vi "Auto_Routine_RightTwoPieceThen2CenterTRAJ.vi"   [LabVIEW 2023]
uses:
  Arm2/ArmGetSetpointEnum.ctl
  Trajectory/TrajectoryGlobals.vi
  <vilib>/Rock Robotics/WPI/ThirdParty/JAS_Junk/TrajLib/Trajectory_Library.lvlib
types:
  T1 = typedef "ArmGetSetpointEnum.ctl" = enum16{"ArmFloorPickup", "ArmAmpDeposit", "ArmSpeakerShoot", "ArmStartPosition", "ArmRestPosition", "ArmSourceIntake", "ArmAwayShoot"}
  T2 = typedef "Trajectory_Library.lvlib/TRAJECTORY.ctl" = cluster{"TotalTImeSecs":dbl, "States":T3[]}
  T3 = typedef "Trajectory_Library.lvlib/TRAJ_STATE.ctl" = cluster{"TimeSeconds":dbl, "Velocity":dbl, "Acceleration":dbl, "POSE":T4, "Curvature":dbl}
  T4 = typedef "Trajectory_Library.lvlib/POSE2D.ctl" = cluster{"TRANSLATION":T5, "ROTATION":T6}
  T5 = typedef "Trajectory_Library.lvlib/TRANSLATION2D.ctl" = cluster{"X":dbl, "Y":dbl}
  T6 = typedef "Trajectory_Library.lvlib/ROTATION2D.ctl" = cluster{"VALUE":dbl, "COS":dbl, "SIN":dbl}
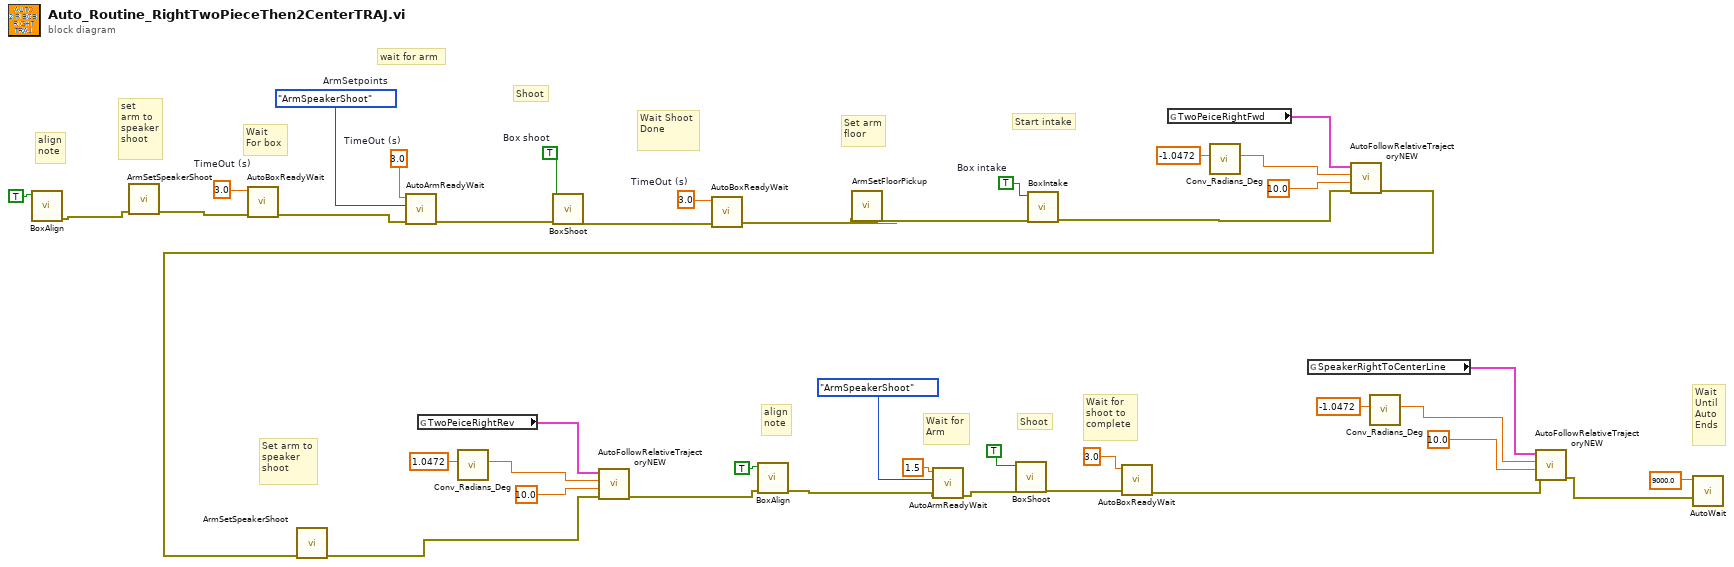
[diagram p0: block diagram]
diagram:
  w31 = 3.0  # TimeOut (s)
  w41 = TRUE  # Box intake
  w40 = TRUE  # Box shoot
  w39 = ArmGetSetpointEnum."ArmSpeakerShoot"  # ArmSetpoints
  w38 = 3.0  # TimeOut (s)
  w34 = 3.0  # TimeOut (s)
  # "align\nnote"
  # "Wait\nUntil\nAuto \nEnds"
  # "Wait for\nshoot to\ncomplete"
  # "Shoot"
  # "Wait for\nArm"
  # "Set arm to\nspeaker \nshoot"
  # "Start intake"
  # "Set arm\nfloor"
  # "Wait Shoot\nDone"
  # "Shoot"
  # "Wait\nFor box"
  # "set \narm to\nspeaker\nshoot"
  # "align\nnote"
  # "wait for arm"
  n1 = call "BoxAlign.vi"("box align"=TRUE) -> ("error out"=w32:errorcluster)  [unwired: 10 in]
  n2 = call "ArmSetSpeakerShoot.vi"("error in (no error)"=w32) -> ("error out"=w30:errorcluster)  [unwired: 10 in]
  n3 = call "AutoBoxReadyWait.vi"("error in (no error)"=w30, "TimeOut (s)"=w31) -> ("error out"=w29:errorcluster)  [unwired: 9 in]
  n4 = call "AutoArmReadyWait.vi"("error in (no error)"=w29, "ArmSetpoints"=w39, "TimeOut (s)"=w38) -> ("error out"=w35:errorcluster)  [unwired: 8 in]
  n5 = global read "TrajectoryGlobals.vi" "TwoPeiceRightRev"() -> (w14:T2)
  n6 = call <vilib>:"Conv_Radians_Deg.vi"("Radians"=1.0472) -> ("Degrees"=w12:dbl)  [unwired: 10 in]
  n7 = call "BoxShoot.vi"("error in (no error)"=w35, "Box shoot"=w40) -> ("error out"=w36:errorcluster)  [unwired: 9 in]
  n8 = call "AutoBoxReadyWait.vi"("error in (no error)"=w36, "TimeOut (s)"=w34) -> ("error out"=w28:errorcluster)  [unwired: 9 in]
  n9 = call "ArmSetFloorPickup.vi"("error in (no error)"=w28) -> ("error out"=w37:errorcluster)  [unwired: 10 in]
  n10 = call "BoxIntake.vi"("error in (no error)"=w37, "Box intake"=w41) -> ("error out"=w27:errorcluster)  [unwired: 9 in]
  n11 = global read "TrajectoryGlobals.vi" "TwoPeiceRightFwd"() -> (w26:T2)
  n12 = call <vilib>:"Conv_Radians_Deg.vi"("Radians"=-1.0472) -> ("Degrees"=w24:dbl)  [unwired: 10 in]
  n13 = global read "TrajectoryGlobals.vi" "SpeakerRightToCenterLine"() -> (w6:T2)
  n14 = call "AutoFollowRelativeTrajectoryNEW.vi"("error in (no error)"=w27, "TimeOut (s)"=10.0, "End Orientation"=w24, "Trajectory"=w26) -> ("error out"=w22:errorcluster)  [unwired: 7 in]
  n15 = call "ArmSetSpeakerShoot.vi"("error in (no error)"=w22) -> ("error out"=w10:errorcluster)  [unwired: 10 in]
  n16 = call "AutoFollowRelativeTrajectoryNEW.vi"("error in (no error)"=w10, "TimeOut (s)"=10.0, "End Orientation"=w12, "Trajectory"=w14) -> ("error out"=w8:errorcluster)  [unwired: 7 in]
  n17 = call "BoxAlign.vi"("error in (no error)"=w8, "box align"=TRUE) -> ("error out"=w7:errorcluster)  [unwired: 9 in]
  n18 = call "AutoArmReadyWait.vi"("error in (no error)"=w7, "ArmSetpoints"=ArmGetSetpointEnum."ArmSpeakerShoot", "TimeOut (s)"=1.5) -> ("error out"=w17:errorcluster)  [unwired: 8 in]
  n19 = call "BoxShoot.vi"("error in (no error)"=w17, "Box shoot"=TRUE) -> ("error out"=w20:errorcluster)  [unwired: 9 in]
  n20 = call "AutoBoxReadyWait.vi"("error in (no error)"=w20, "TimeOut (s)"=3.0) -> ("error out"=w2:errorcluster)  [unwired: 9 in]
  n21 = call <vilib>:"Conv_Radians_Deg.vi"("Radians"=-1.0472) -> ("Degrees"=w4:dbl)  [unwired: 10 in]
  n22 = call "AutoFollowRelativeTrajectoryNEW.vi"("error in (no error)"=w2, "TimeOut (s)"=10.0, "End Orientation"=w4, "Trajectory"=w6) -> ("error out"=w1:errorcluster)  [unwired: 7 in]
  n23 = call "AutoWait.vi"("error in (no error)"=w1, "TimeOut (s)"=9000.0) -> ()  [unwired: 9 in, 1 out]
